vi "STS_Add_Ref_MPMData_CH.vi"(8 "错误输入（无错误）":errorcluster, 9 "data":sgl[](array[numeric]), 10 "STSProcess.ILSTS":refnum<k24>, 11 "Setting":refnum<k24>) -> (0 "错误输出":errorcluster, 3 "ILSTS":refnum<k24>)   [LabVIEW 2017]
doc: "Add in to MPM reference data to STS Process Class"
uses:
  D:/test/ILSTS/LV_IL/LV_IL_Sample_x64/DLL/STSProcess.dll
  DLL/STSProcess.dll
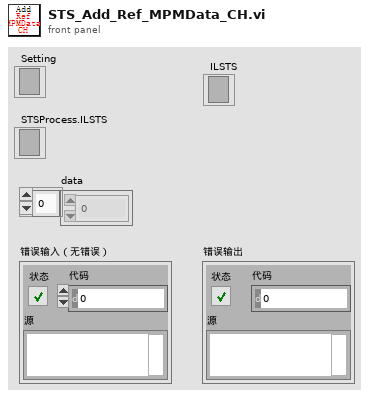
[diagram p1: front panel]
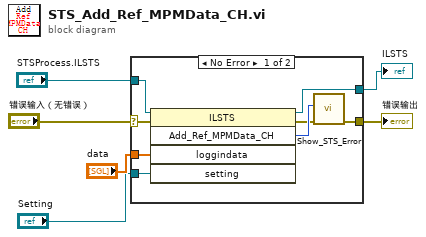
[diagram p0: block diagram]
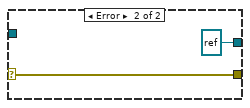
[diagram p2: hidden frame]
diagram:
  n1 = case shown="No Error" "错误输入（无错误）" {
    selector: "错误输入（无错误）" -> [w11 w16]
    tunnel: [w7 w16] -> w6
    tunnel: "data" -> [w14 _]
    tunnel: "Setting" -> [w13 _]
    tunnel: "STSProcess.ILSTS" -> [w12 _]
    tunnel: [w10 refnum<k24> refnum ("STSProcess.ILSTS")] -> w1
    frame No Error {
      n2 = invoke on="调用节点" class="ILSTS" method="Add_Ref_MPMData_CH"(reference=w12, error in=w11, "loggindata"=w14, "setting"=w13) -> (reference out=w10:refnum<k24>, error out=w8:errorcluster, "Add_Ref_MPMData_CH"=w9:i32)  [unwired: 1 in, 2 out]
      n3 = call "Show_STS_Error.vi"("error in (no error)"=w8, "Error"=w9) -> ("error out"=w7:errorcluster)  [unwired: 9 in]
    }
    frame Error {
    }
  }
  "错误输出" <- w6
  "ILSTS" <- w1
